vi "Parse Rx Label Buffer Read Outputs.vi"(10 "px_Info out":cluster{"ixw":u16, "inr":u16, "ci":u16}, 11 "px_LData":u32[](array[numeric])) -> (0 "receiving error":bool, 1 "hit":bool, 2 "time stamp":dbl, 3 "data word":u32 format="%032b", 4 "specific errors":T1)   [LabVIEW 2024, in "AIM ARINC 429 Hardware API.lvlib"]
uses:
  AIM ARINC 429 Hardware API.lvlib
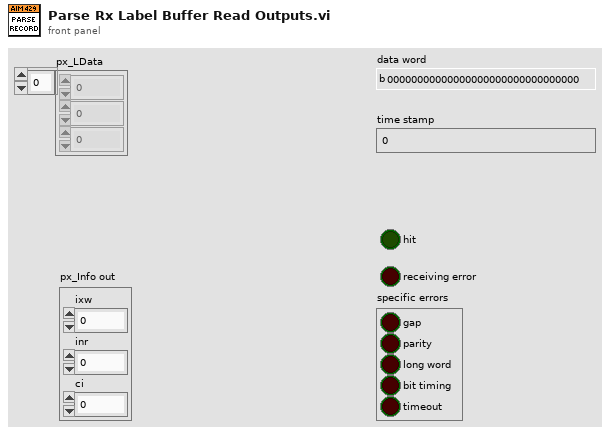
[diagram p1: front panel]
types:
  T1 = cluster{"gap":bool, "parity":bool, "long word":bool, "bit timing":bool, "timeout":bool}
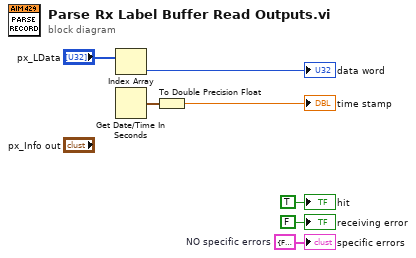
[diagram p0: block diagram]
diagram:
  w1 = T1 {"gap"=FALSE, "parity"=FALSE, "long word"=FALSE, "bit timing"=FALSE, "timeout"=FALSE}  # NO specific errors
  n1 = Index Array(array="px_LData") -> (element=→"data word":u32)  [unwired: 1 in]
  n2 = Get Date/Time In Seconds() -> (seconds since 1Jan1904=w7:timestamp)
  n3 = To Double Precision Float(number=w7) -> (double precision float=→"time stamp":dbl)
  "specific errors" <- w1
  "hit" <- TRUE ("hit")
  "receiving error" <- FALSE ("receiving error")
